vi "InclinometerLogic.vi"   [LabVIEW 2016]
uses:
  InclinometerData.ctl
  InclinometerStates.ctl
  <vilib>/Platform/TimedLoop/XDataNode/timing_clust.ctl
  <vilib>/Platform/TimedLoop/XDataNode/nitl_modes.ctl
  <vilib>/Platform/TimedLoop/XDataNode/wakeup.ctl
  Telemetry/TelemetryFields.ctl
  Telemetry/TelemetryDataTypes.ctl
  Telemetry/TelemetryUpdateModes.ctl
  InclinometerErrorCodes.ctl
  <vilib>/rvi/Emulation/niFpgaSctlEmulationGetInTimedLoop.vi
  <vilib>/rvi/Emulation/niFpgaEmulationReportErrorSimple.vi
  <vilib>/rvi/Emulation/niFpgaGetClockAttributes.vi
  <vilib>/rvi/Emulation/niFpgaCriticalErrorInLSC.vi
  <vilib>/rvi/Emulation/niFpgaEmulationIsFPGAContextNoSignature.vi
  <vilib>/rvi/DataTransferAndStorage/Container/Common/niFpgaContainerGetUniqueNameForEmu.vi
  <vilib>/rvi/Memory/Memory_Emulation/niFpgaMemoryEmulationCacheClearOnFirstRun.vi
  <vilib>/rvi/Memory/Memory_Emulation/nirvimemoryEmulationManagerCache_MakeExclusive.vi
  <vilib>/rvi/Memory/Memory_Emulation/niFpgaMemoryEmulationValidateCache.vi
  <vilib>/rvi/Memory/Memory_Emulation/nirvimemoryEmulationManagerCache_InsertValue.vi
  <vilib>/Utility/error.llb/Clear Errors.vi
  <vilib>/rvi/Memory/Memory_Emulation/nirvimemoryEmulationManagerCache_ReleaseExclusive.vi
  <vilib>/rvi/Memory/Memory_Emulation/nirvimemoryEmulationManagerCache_GetValue.vi
  <vilib>/rvi/Memory/Memory_Emulation/nirvimemoryEmulationManagerCache_SetValue.vi
  <vilib>/rvi/Emulation/niFpgaProcessEmulError.vi
  <vilib>/rvi/errors/niFpgaSetErrorForExecOnDevCompSimple.vi
  <vilib>/rvi/eio/common/nirviEmuReportErrorAndStop.vi
  <vilib>/rvi/FIFO/Fifo_Resource/nirvififoEmulationSetSize.vi
  <vilib>/rvi/FIFO/Fifo_Resource/nirviFifoEmulationQueueMgr.vi
  <instcachedir>/0/nirviFifoEmulationQueueMgr_E5CAEC123FF24DC58D834DCA3CDAA9B5.lvgen/nirviFifoEmulationQueueMgr_E5CAEC123FF24DC58D834DCA3CDAA9B5_004.vi
  <vilib>/rvi/FIFO/Fifo_Resource/nirvififoEmulationDetermineInputValidOut.vi
  <vilib>/rvi/FIFO/Fifo_Resource/nirvififoEmulationCreateLock.vi
  <vilib>/rvi/FIFO/Fifo_Resource/nirvififoEmulationObtainLock.vi
  <vilib>/rvi/FIFO/Fifo_Resource/nirvififoEmulationReleaseLock.vi
  <vilib>/rvi/occurrence/nirviWaitOnOccurrenceBase.vi
  <vilib>/rvi/errors/nirviReportUnexpectedCaseInternalError.vi
  <vilib>/rvi/errors/nirviReportUnexpectedCaseInternalError (U32).vi
  <instcachedir>/0/nirviFifoEmulationQueueMgr_E5CAEC123FF24DC58D834DCA3CDAA9B5.lvgen/nirviFifoEmulationQueueMgr_E5CAEC123FF24DC58D834DCA3CDAA9B5_009.vi
  <instcachedir>/0/nirviFifoEmulationQueueMgr_E5CAEC123FF24DC58D834DCA3CDAA9B5.lvgen/nirviFifoEmulationQueueMgr_E5CAEC123FF24DC58D834DCA3CDAA9B5_002.vi
  <instcachedir>/0/nirviFifoEmulationQueueMgr_E5CAEC123FF24DC58D834DCA3CDAA9B5.lvgen/nirviFifoEmulationQueueMgr_E5CAEC123FF24DC58D834DCA3CDAA9B5_024.vi
  <vilib>/rvi/eio/common/nirviEmuTemplateMethod_errors.vi
  <vilib>/Platform/TimedLoop/XDataNode/XDataNode.xnode
  <vilib>/rvi/DataTransferAndStorage/Container/XNode/niFpgaContainer.xnode
  <vilib>/rvi/DataTransferAndStorage/Register/Emulation/niFpgaRegisterEmulation.vi
  <vilib>/rvi/FIFO/Fifo_Resource/nirvififoEmulationWrite.vi
  <vilib>/rvi/FIFO/Fifo_Resource/nirvififoEmulationRead.vi
  <vilib>/eio/EIONode/EIONode.xnode
  <vilib>/Platform/TimedLoop/XDataNode/XDNodeRunTimeDep.lvlib
types:
  T1 = typedef "InclinometerData.ctl" = cluster{"InclinometerState":T2, "Timestamp":u64, "Timeout":i32, "Angle":u32, "CRC":u16, "Exception":u8}
  T2 = typedef "InclinometerStates.ctl" = enum16{"WaitForTrigger", "ClearRxFIFO", "WaitForClearComplete", "WriteAddress", "WriteFunction", "WriteStartAddress1", "WriteStartAddress0", "WriteAddressCount1", "WriteAddressCount0", "WriteCRC1", "WriteCRC0", "ReadAddress", "ReadFunction", "ReadByteCount", "ReadDataByte1", "ReadDataByte0", "ReadDataByte3", "ReadDataByte2", "ReadCRCByte0", "ReadCRCByte1", "CalculateCRC", "ValidateCRC", "MoveTimestamp", "MoveData", "ClearErrorCode", "ReadExceptionCode", "ReadExceptionCRCByte0", "ReadExceptionCRCByte1", "CalculateExceptionCRC", "ValidateExceptionCRC", "ParseExceptionCode", "ResponseAddressError", "ResponseFunctionCodeError", "ResponseByteCountError", "ResponseCRCError", "ResponseUnknownError", "ResponseTimeoutError", "SensorReportsIllegalFunction", "SensorReportsIllegalDataAddress"}
  T3 = typedef "XDNodeRunTimeDep.lvlib/timing_clust.ctl" = cluster{"Expected End [f-1]":u64, "Actual End [f-1]":u64, "Finished Late? [f-1]":bool, "Expected End [i-1]":u64, "Actual End [i-1]":u64, "Finished Late? [i-1]":bool, "Expected Start [i]":u64, "Actual Start [i]":u64, "Expected Start [f]":u64, "Actual Start [f]":u64, "Source Name":string, "Structure Name":string, "Period":i64, "Deadline":i64, "Offset":i64, "Start":i64, "Priority":i32, "Timeout":i32, "Mode":T4, "Wakeup Reason":T5, "Error":errorcluster, "Source Type":string, "Secondary Source Type":string, "Global End Time":u64, "Global Start Time":u64, "Frame Duration":u64, "Iteration Duration":u64, "Assigned CPU":i32, "I/O Scan Engine Mode":u32}
  T4 = typedef "XDNodeRunTimeDep.lvlib/nitl_modes.ctl" = enum32{"No Change", "Process missed periods, maintain original phase", "Discard missed periods, maintain original phase", "Process missed periods, ignore original phase", "Discard missed periods, ignore original phase"}
  T5 = typedef "XDNodeRunTimeDep.lvlib/wakeup.ctl" = enum32{"Normal", "Aborted", "Asynchronous wakeup", "Timing source error", "Timed loop error", "Timeout"}
  T6 = typedef "TelemetryUpdateModes.ctl" = enum8{"=", "+", "-", "|"}
  T7 = typedef "TelemetryDataTypes.ctl" = enum8{"U8", "U16", "U32", "U64", "I8", "I16", "I32", "I64", "SGL"}
  T8 = typedef "TelemetryFields.ctl" = enum16{"InclinometerErrorCode", "InclinometerTxBytes", "InclinometerRxBytes", "InclinometerTxFrames", "InclinometerRxFrames", "InclinometerTimestamp", "InclinometerAngle", "DisplacementErrorCode", "DisplacementTxBytes", "DisplacementRxBytes", "DisplacementTxFrames", "DisplacementRxFrames", "DisplacementTimestamp", "Displacement1", "Displacement2", "Displacement3", "Displacement4", "Displacement5", "Displacement6", "Displacement7", "Displacement8", "AccelerometerSampleCount", "AccelerometerTimestamp", "AccelerometerRaw1", "AccelerometerRaw2", "AccelerometerRaw3", "AccelerometerRaw4", "AccelerometerRaw5", "AccelerometerRaw6", "AccelerometerRaw7", "AccelerometerRaw8", "AccelerometerEng1", "AccelerometerEng2", "AccelerometerEng3", "AccelerometerEng4", "AccelerometerEng5", "AccelerometerEng6", "AccelerometerEng7", "AccelerometerEng8", "AngularAccelerationX", "AngularAccelerationY", "AngularAccelerationZ"}
  T9 = typedef "InclinometerErrorCodes.ctl" = enum8{"None", "ResponseAddressError", "ResponseFunctionCodeError", "ResponseByteCountError", "ResponseCRCError", "ResponseUnknownError", "ResponseTimeoutError", "SensorReportsIllegalFunction", "SensorReportsIllegalDataAddress"}
  T10 = typedef "TelemetryUpdateData.ctl" = cluster{"DataType":T7, "Mode":T6, "Field":T8, "Data":u64}
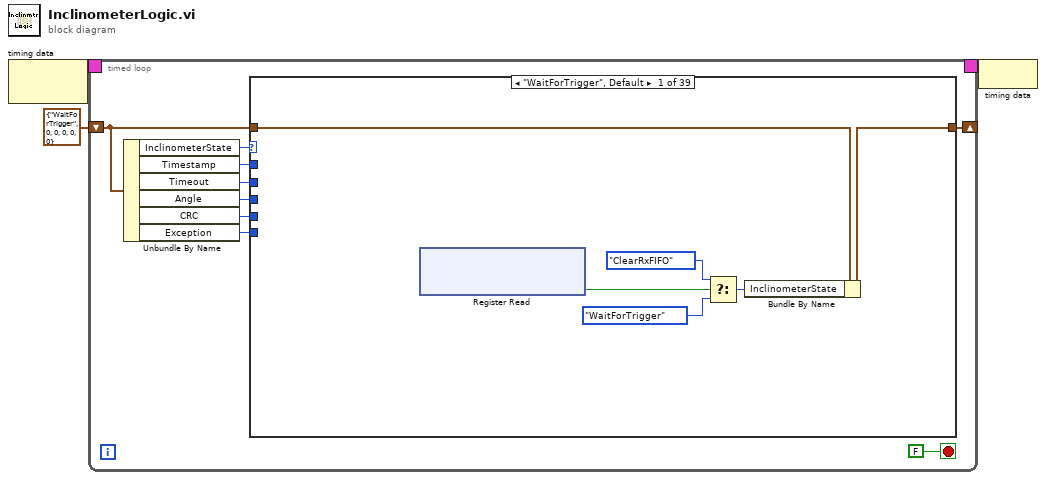
[diagram p0: block diagram]
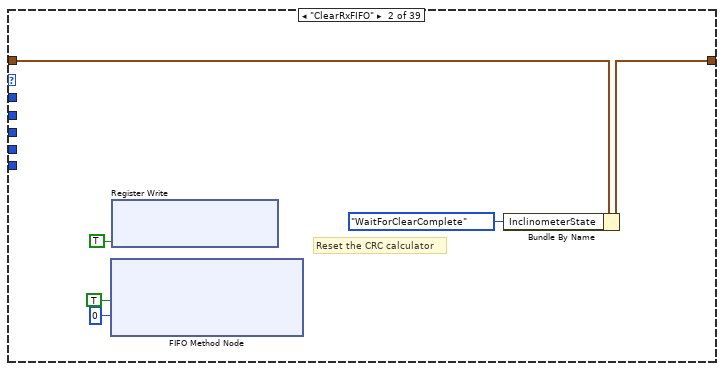
[diagram p2: hidden frame]
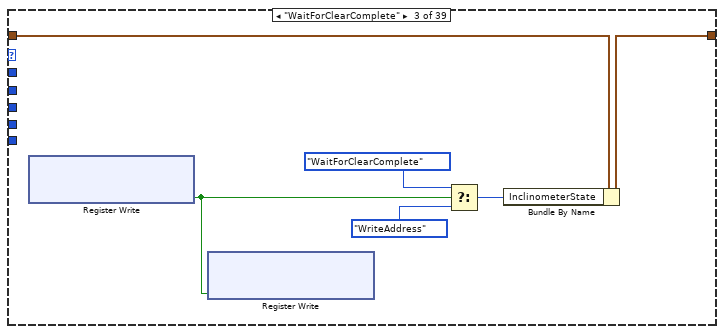
[diagram p3: hidden frame]
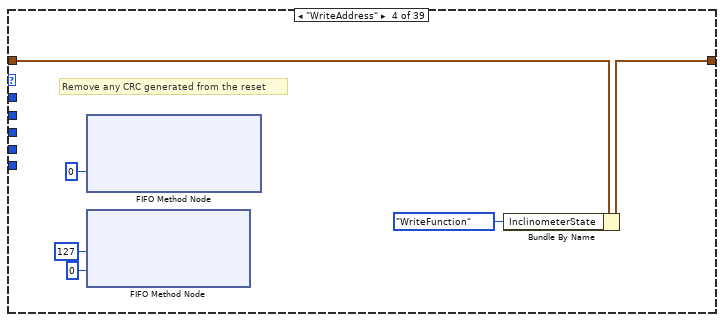
[diagram p4: hidden frame]
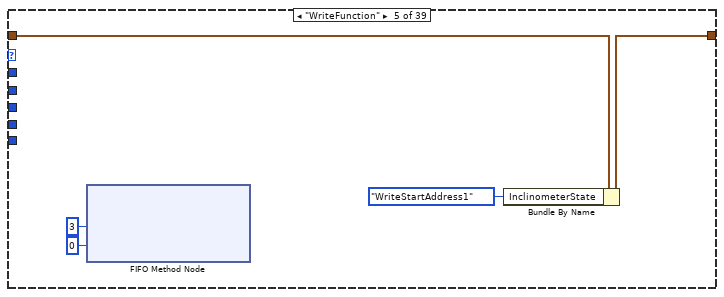
[diagram p5: hidden frame]
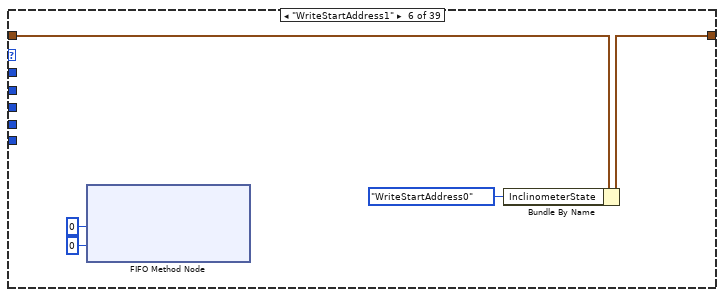
[diagram p6: hidden frame]
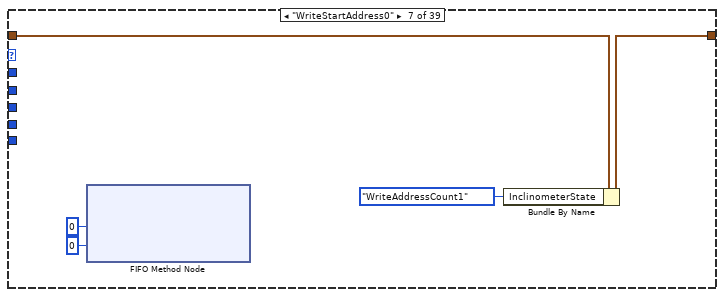
[diagram p7: hidden frame]
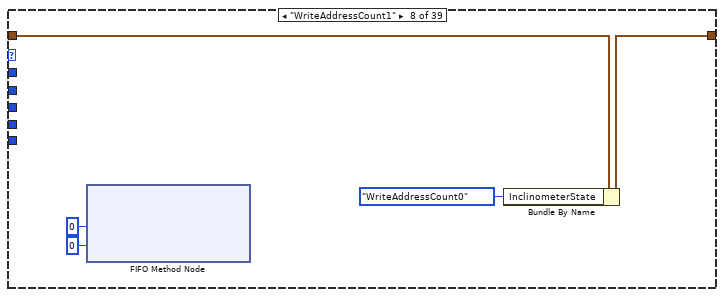
[diagram p8: hidden frame]
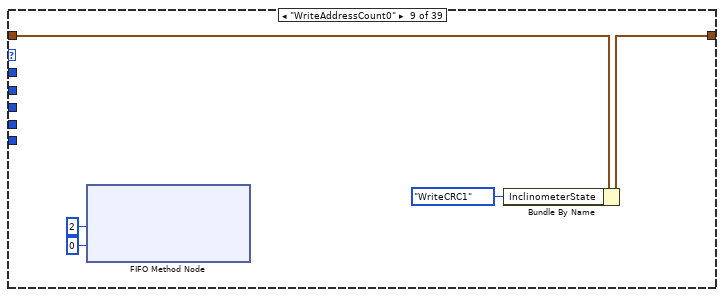
[diagram p9: hidden frame]
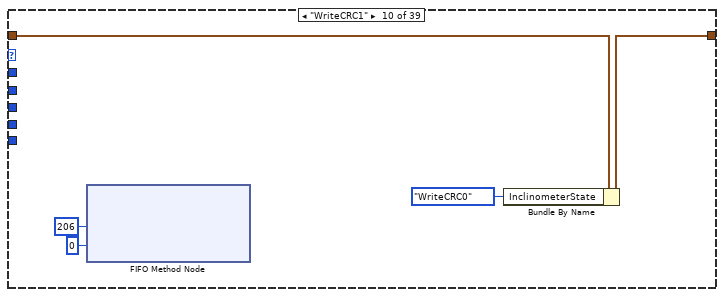
[diagram p10: hidden frame]
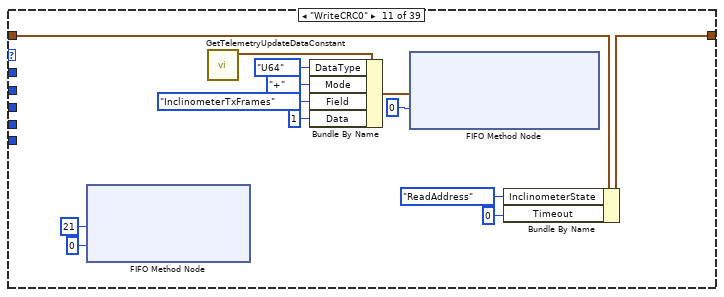
[diagram p11: hidden frame]
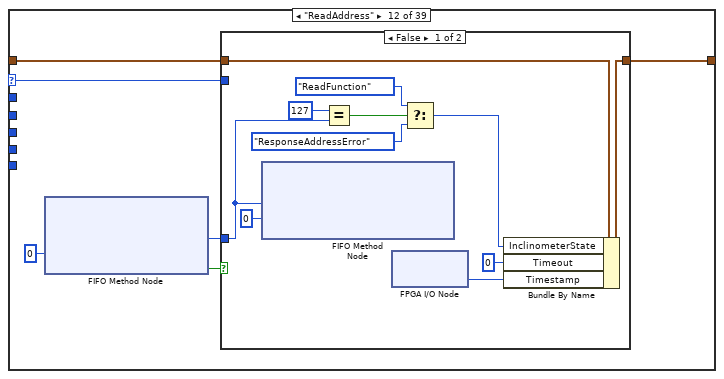
[diagram p12: hidden frame]
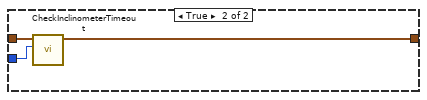
[diagram p13: hidden frame]
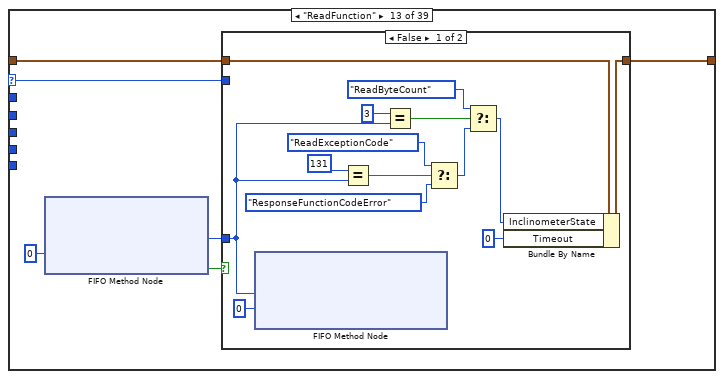
[diagram p14: hidden frame]
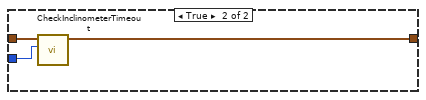
[diagram p15: hidden frame]
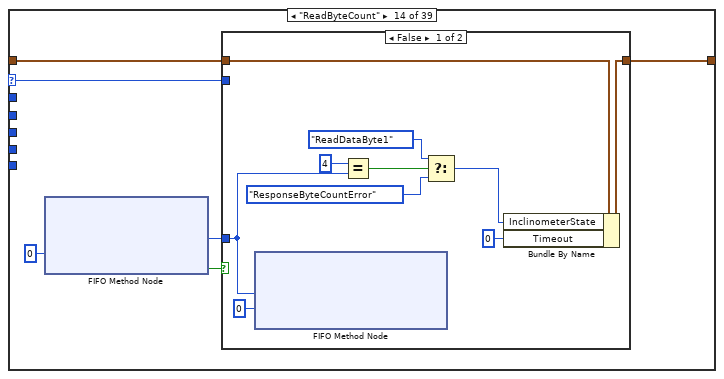
[diagram p16: hidden frame]
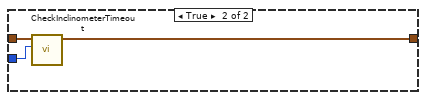
[diagram p17: hidden frame]
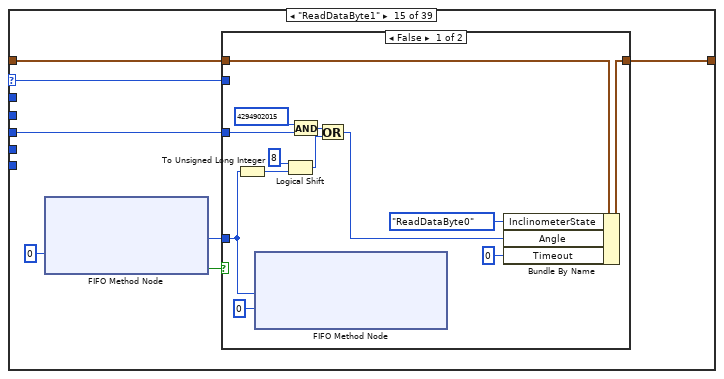
[diagram p18: hidden frame]
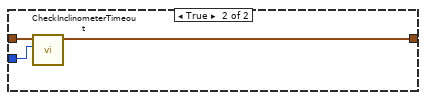
[diagram p19: hidden frame]
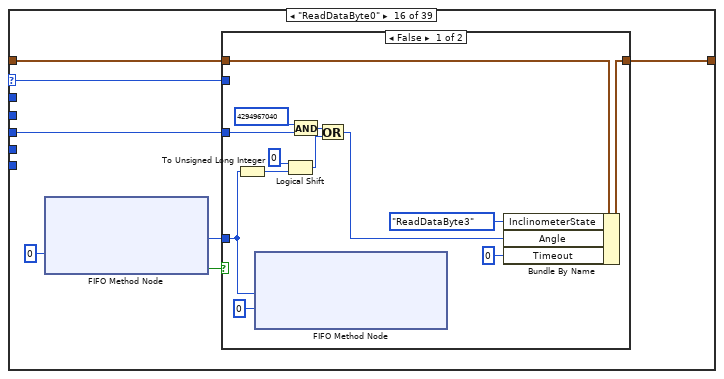
[diagram p20: hidden frame]
diagram:
  n1 = node-c288() -> (w3:T3)  [unwired: 1 in]
  n2 = timed-loop {
    timing: w3 -> [_]
    timing-out: [_] -> w2
    shift-right: [w11] -> _
    shift-left: T1 {"InclinometerState"=enum."WaitForTrigger", "Timestamp"=0, "Timeout"=0, "Angle"=0, "CRC"=0, "Exception"=0} ("InclinometerData") -> [w12]
    stop <- FALSE stop-if-true
    n3 = Unbundle By Name(w12) -> ("InclinometerState"=w10:T2, "Timestamp"=w5:u64, "Timeout"=w9:i32, "Angle"=w8:u32, "CRC"=w7:u16, "Exception"=w4:u8)
    n4 = case shown="\"WaitForTrigger\", Default" w10 {
      selector: w10 -> [_ _ _ _ _ _ _ _ _ _ _ w80 w100 w123 w142 w165 w188 w211 w234 w256 _ _ _ _ _ w335 w357 w379 _ _ _ _ _ _ _ _ _ _ _]
      tunnel: w12 -> [w17 w23 w29 w35 w40 w45 w50 w55 w60 w65 w78 w81 w101 w124 w144 w167 w190 w213 w236 w258 w281 w284 w313 w323 w333 w336 w359 w381 w404 w407 w434 w444 w454 w464 w474 w484 w494 w504 w514]
      tunnel: [w18 w24 w30 w36 w41 w46 w51 w56 w61 w66 w79 w82 w102 w125 w145 w168 w191 w214 w237 w259 w282 w285 w314 w324 w334 w337 w360 w382 w405 w408 w435 w445 w455 w465 w475 w485 w495 w505 w515] -> w11
      tunnel: w9 -> [_ _ _ _ _ _ _ _ _ _ _ _ _ _ _ _ _ _ _ _ _ _ _ _ _ _ _ _ _ _ _ _ _ _ _ _ _ _ _]
      tunnel: w8 -> [_ _ _ _ _ _ _ _ _ _ _ _ _ _ w143 w166 w189 w212 _ _ _ _ _ w315 _ _ _ _ _ _ _ _ _ _ _ _ _ _ _]
      tunnel: w7 -> [_ _ _ _ _ _ _ _ _ _ _ _ _ _ _ _ _ _ w235 w257 _ w283 _ _ _ _ w358 w380 _ w406 _ _ _ _ _ _ _ _ _]
      tunnel: w5 -> [_ _ _ _ _ _ _ _ _ _ _ _ _ _ _ _ _ _ _ _ _ _ w305 _ _ _ _ _ _ _ _ _ _ _ _ _ _ _ _]
      tunnel: w4 -> [_ _ _ _ _ _ _ _ _ _ _ _ _ _ _ _ _ _ _ _ _ _ _ _ _ _ _ _ _ _ w429 _ _ _ _ _ _ _ _]
      frame "WaitForTrigger", Default {
        n5 = xnode ("Register Read")() -> ("Data"=w13:bool)  [unwired: 1 in, 1 out]
        n6 = Select(t=InclinometerStates."ClearRxFIFO" ("InclinometerState"), s=w13, f=InclinometerStates."WaitForTrigger" ("InclinometerState")) -> (s? t:f=w14:T2)
        n7 = Bundle By Name(cluster=w17, "InclinometerState"=w14) -> (w18:T1)
      }
      frame "ClearRxFIFO" {
        # "Reset the CRC calculator"
        n8 = xnode ("FIFO Method Node")("Element"=TRUE, "Timeout"=0) -> ()  [unwired: 1 in, 2 out]
        n9 = xnode ("Register Write")("Data"=TRUE) -> ()  [unwired: 1 in, 1 out]
        n10 = Bundle By Name(cluster=w23, "InclinometerState"=InclinometerStates."WaitForClearComplete") -> (w24:T1)
      }
      frame "WaitForClearComplete" {
        n11 = xnode ("Register Write")() -> ("Data"=w25:bool)  [unwired: 1 in, 1 out]
        n12 = xnode ("Register Write")("Data"=w25) -> ()  [unwired: 1 in, 1 out]
        n13 = Select(t=InclinometerStates."WaitForClearComplete", s=w25, f=InclinometerStates."WriteAddress" ("InclinometerState")) -> (s? t:f=w26:T2)
        n14 = Bundle By Name(cluster=w29, "InclinometerState"=w26) -> (w30:T1)
      }
      frame "WriteAddress" {
        # "Remove any CRC generated from the reset"
        n15 = xnode ("FIFO Method Node")("Timeout"=0) -> ()  [unwired: 1 in, 3 out]
        n16 = xnode ("FIFO Method Node")("Element"=u8 127, "Timeout"=0) -> ()  [unwired: 1 in, 2 out]
        n17 = Bundle By Name(cluster=w35, "InclinometerState"=InclinometerStates."WriteFunction") -> (w36:T1)
      }
      frame "WriteFunction" {
        n18 = xnode ("FIFO Method Node")("Element"=u8 3, "Timeout"=0) -> ()  [unwired: 1 in, 2 out]
        n19 = Bundle By Name(cluster=w40, "InclinometerState"=InclinometerStates."WriteStartAddress1") -> (w41:T1)
      }
      frame "WriteStartAddress1" {
        n20 = xnode ("FIFO Method Node")("Element"=u8 0, "Timeout"=0) -> ()  [unwired: 1 in, 2 out]
        n21 = Bundle By Name(cluster=w45, "InclinometerState"=InclinometerStates."WriteStartAddress0") -> (w46:T1)
      }
      frame "WriteStartAddress0" {
        n22 = xnode ("FIFO Method Node")("Element"=u8 0, "Timeout"=0) -> ()  [unwired: 1 in, 2 out]
        n23 = Bundle By Name(cluster=w50, "InclinometerState"=InclinometerStates."WriteAddressCount1") -> (w51:T1)
      }
      frame "WriteAddressCount1" {
        n24 = xnode ("FIFO Method Node")("Element"=u8 0, "Timeout"=0) -> ()  [unwired: 1 in, 2 out]
        n25 = Bundle By Name(cluster=w55, "InclinometerState"=InclinometerStates."WriteAddressCount0") -> (w56:T1)
      }
      frame "WriteAddressCount0" {
        n26 = xnode ("FIFO Method Node")("Element"=u8 2, "Timeout"=0) -> ()  [unwired: 1 in, 2 out]
        n27 = Bundle By Name(cluster=w60, "InclinometerState"=InclinometerStates."WriteCRC1") -> (w61:T1)
      }
      frame "WriteCRC1" {
        n28 = xnode ("FIFO Method Node")("Element"=u8 206, "Timeout"=0) -> ()  [unwired: 1 in, 2 out]
        n29 = Bundle By Name(cluster=w65, "InclinometerState"=InclinometerStates."WriteCRC0") -> (w66:T1)
      }
      frame "WriteCRC0" {
        n30 = xnode ("FIFO Method Node")("Element"=u8 21, "Timeout"=0) -> ()  [unwired: 1 in, 2 out]
        n31 = call "GetTelemetryUpdateDataConstant.vi"() -> ("TelemetryUpdateData"=w71:T10)  [unwired: 11 in]
        n32 = Bundle By Name(cluster=w71, "DataType"=TelemetryDataTypes."U64" ("TelemetryDataTypes"), "Mode"=TelemetryUpdateModes."+" ("TelemetryUpdateModes"), "Field"=TelemetryFields."InclinometerTxFrames", "Data"=u64 1) -> (w67:T10)
        n33 = xnode ("FIFO Method Node")("Element"=w67, "Timeout"=0) -> ()  [unwired: 1 in, 2 out]
        n34 = Bundle By Name(cluster=w78, "InclinometerState"=InclinometerStates."ReadAddress", "Timeout"=0) -> (w79:T1)
      }
      frame "ReadAddress" {
        n35 = xnode ("FIFO Method Node")("Timeout"=0) -> ("Element"=w83:u8, "Timed Out?"=w84:bool)  [unwired: 1 in, 1 out]
        n36 = case shown="False" w84 {
          tunnel: w83 -> [w93 _]
          tunnel: [w95 w98] -> w82
          tunnel: w81 -> [w96 w99]
          tunnel: w80 -> [_ w97]
          frame False {
            n37 = xnode ("FIFO Method Node")("Element"=w93, "Timeout"=0) -> ()  [unwired: 1 in, 2 out]
            n38 = Equal?(x=u8 127, y=w93) -> (x = y?=w91:bool)
            n39 = xnode "FPGA I/O Node"() -> ("Time"=w86:u64)  [unwired: 1 in, 1 out]
            n40 = Select(t=InclinometerStates."ReadFunction" ("InclinometerState"), s=w91, f=InclinometerStates."ResponseAddressError" ("InclinometerState")) -> (s? t:f=w88:T2)
            n41 = Bundle By Name(cluster=w96, "InclinometerState"=w88, "Timeout"=0, "Timestamp"=w86) -> (w95:T1)
          }
          frame True {
            n42 = call "CheckInclinometerTimeout.vi"("StateIfNoTimeout"=w97, "InclinometerData in"=w99) -> ("InclinometerData out"=w98:T1)  [unwired: 9 in]
          }
        }
      }
      frame "ReadFunction" {
        n43 = xnode ("FIFO Method Node")("Timeout"=0) -> ("Element"=w103:u8, "Timed Out?"=w104:bool)  [unwired: 1 in, 1 out]
        n44 = case shown="False" w104 {
          tunnel: w103 -> [w111 _]
          tunnel: [w118 w121] -> w102
          tunnel: w101 -> [w119 w122]
          tunnel: w100 -> [_ w120]
          frame False {
            n45 = xnode ("FIFO Method Node")("Element"=w111, "Timeout"=0) -> ()  [unwired: 1 in, 2 out]
            n46 = Equal?(x=u8 131, y=w111) -> (x = y?=w110:bool)
            n47 = Equal?(x=u8 3, y=w111) -> (x = y?=w115:bool)
            n48 = Select(t=InclinometerStates."ReadExceptionCode" ("InclinometerState"), s=w110, f=InclinometerStates."ResponseFunctionCodeError" ("InclinometerState")) -> (s? t:f=w113:T2)
            n49 = Select(t=InclinometerStates."ReadByteCount" ("InclinometerState"), s=w115, f=w113) -> (s? t:f=w107:T2)
            n50 = Bundle By Name(cluster=w119, "InclinometerState"=w107, "Timeout"=0) -> (w118:T1)
          }
          frame True {
            n51 = call "CheckInclinometerTimeout.vi"("StateIfNoTimeout"=w120, "InclinometerData in"=w122) -> ("InclinometerData out"=w121:T1)  [unwired: 9 in]
          }
        }
      }
      frame "ReadByteCount" {
        n52 = xnode ("FIFO Method Node")("Timeout"=0) -> ("Element"=w126:u8, "Timed Out?"=w127:bool)  [unwired: 1 in, 1 out]
        n53 = case shown="False" w127 {
          tunnel: w126 -> [w135 _]
          tunnel: [w137 w140] -> w125
          tunnel: w124 -> [w138 w141]
          tunnel: w123 -> [_ w139]
          frame False {
            n54 = xnode ("FIFO Method Node")("Element"=w135, "Timeout"=0) -> ()  [unwired: 1 in, 2 out]
            n55 = Equal?(x=u8 4, y=w135) -> (x = y?=w133:bool)
            n56 = Select(t=InclinometerStates."ReadDataByte1" ("InclinometerState"), s=w133, f=InclinometerStates."ResponseByteCountError" ("InclinometerState")) -> (s? t:f=w130:T2)
            n57 = Bundle By Name(cluster=w138, "InclinometerState"=w130, "Timeout"=0) -> (w137:T1)
          }
          frame True {
            n58 = call "CheckInclinometerTimeout.vi"("StateIfNoTimeout"=w139, "InclinometerData in"=w141) -> ("InclinometerData out"=w140:T1)  [unwired: 9 in]
          }
        }
      }
      frame "ReadDataByte1" {
        n59 = xnode ("FIFO Method Node")("Timeout"=0) -> ("Element"=w146:u8, "Timed Out?"=w147:bool)  [unwired: 1 in, 1 out]
        n60 = case shown="False" w147 {
          tunnel: w146 -> [w152 _]
          tunnel: [w160 w163] -> w145
          tunnel: w144 -> [w161 w164]
          tunnel: w143 -> [w156 _]
          tunnel: w142 -> [_ w162]
          frame False {
            n61 = To Unsigned Long Integer(number=w152) -> (unsigned 32bit integer=w151:u32)
            n62 = xnode ("FIFO Method Node")("Element"=w152, "Timeout"=0) -> ()  [unwired: 1 in, 2 out]
            n63 = Logical Shift(y=i16 8, x=w151) -> (x << y=w154:u32)
            n64 = And(x=u32 4294902015, y=w156) -> (x .and. y?=w153:u32)
            n65 = Or(x=w153, y=w154) -> (x .or. y?=w150:u32)
            n66 = Bundle By Name(cluster=w161, "InclinometerState"=InclinometerStates."ReadDataByte0", "Angle"=w150, "Timeout"=0) -> (w160:T1)
          }
          frame True {
            n67 = call "CheckInclinometerTimeout.vi"("StateIfNoTimeout"=w162, "InclinometerData in"=w164) -> ("InclinometerData out"=w163:T1)  [unwired: 9 in]
          }
        }
      }
      frame "ReadDataByte0" {
        n68 = xnode ("FIFO Method Node")("Timeout"=0) -> ("Element"=w169:u8, "Timed Out?"=w170:bool)  [unwired: 1 in, 1 out]
        n69 = case shown="False" w170 {
          tunnel: w169 -> [w175 _]
          tunnel: [w183 w186] -> w168
          tunnel: w167 -> [w184 w187]
          tunnel: w166 -> [w179 _]
          tunnel: w165 -> [_ w185]
          frame False {
            n70 = To Unsigned Long Integer(number=w175) -> (unsigned 32bit integer=w174:u32)
            n71 = xnode ("FIFO Method Node")("Element"=w175, "Timeout"=0) -> ()  [unwired: 1 in, 2 out]
            n72 = Logical Shift(y=i16 0, x=w174) -> (x << y=w177:u32)
            n73 = And(x=u32 4294967040, y=w179) -> (x .and. y?=w176:u32)
            n74 = Or(x=w176, y=w177) -> (x .or. y?=w173:u32)
            n75 = Bundle By Name(cluster=w184, "InclinometerState"=InclinometerStates."ReadDataByte3", "Angle"=w173, "Timeout"=0) -> (w183:T1)
          }
          frame True {
            n76 = call "CheckInclinometerTimeout.vi"("StateIfNoTimeout"=w185, "InclinometerData in"=w187) -> ("InclinometerData out"=w186:T1)  [unwired: 9 in]
          }
        }
      }
      frame "ReadDataByte3" {
        n77 = xnode ("FIFO Method Node")("Timeout"=0) -> ("Element"=w192:u8, "Timed Out?"=w193:bool)  [unwired: 1 in, 1 out]
        n78 = case shown="False" w193 {
          tunnel: w192 -> [w198 _]
          tunnel: [w206 w209] -> w191
          tunnel: w190 -> [w207 w210]
          tunnel: w189 -> [w202 _]
          tunnel: w188 -> [_ w208]
          frame False {
            n79 = To Unsigned Long Integer(number=w198) -> (unsigned 32bit integer=w197:u32)
            n80 = xnode ("FIFO Method Node")("Element"=w198, "Timeout"=0) -> ()  [unwired: 1 in, 2 out]
            n81 = Logical Shift(y=i16 24, x=w197) -> (x << y=w200:u32)
            n82 = And(x=u32 16777215, y=w202) -> (x .and. y?=w199:u32)
            n83 = Or(x=w199, y=w200) -> (x .or. y?=w196:u32)
            n84 = Bundle By Name(cluster=w207, "InclinometerState"=InclinometerStates."ReadDataByte2", "Angle"=w196, "Timeout"=0) -> (w206:T1)
          }
          frame True {
            n85 = call "CheckInclinometerTimeout.vi"("StateIfNoTimeout"=w208, "InclinometerData in"=w210) -> ("InclinometerData out"=w209:T1)  [unwired: 9 in]
          }
        }
      }
      frame "ReadDataByte2" {
        n86 = xnode ("FIFO Method Node")("Timeout"=0) -> ("Element"=w215:u8, "Timed Out?"=w216:bool)  [unwired: 1 in, 1 out]
        n87 = case shown="False" w216 {
          tunnel: w215 -> [w221 _]
          tunnel: [w229 w232] -> w214
          tunnel: w213 -> [w230 w233]
          tunnel: w212 -> [w225 _]
          tunnel: w211 -> [_ w231]
          frame False {
            n88 = To Unsigned Long Integer(number=w221) -> (unsigned 32bit integer=w220:u32)
            n89 = xnode ("FIFO Method Node")("Element"=w221, "Timeout"=0) -> ()  [unwired: 1 in, 2 out]
            n90 = Logical Shift(y=i16 16, x=w220) -> (x << y=w223:u32)
            n91 = And(x=u32 4278255615, y=w225) -> (x .and. y?=w222:u32)
            n92 = Or(x=w222, y=w223) -> (x .or. y?=w219:u32)
            n93 = Bundle By Name(cluster=w230, "InclinometerState"=InclinometerStates."ReadCRCByte0", "Angle"=w219, "Timeout"=0) -> (w229:T1)
          }
          frame True {
            n94 = call "CheckInclinometerTimeout.vi"("StateIfNoTimeout"=w231, "InclinometerData in"=w233) -> ("InclinometerData out"=w232:T1)  [unwired: 9 in]
          }
        }
      }
      frame "ReadCRCByte0" {
        n95 = xnode ("FIFO Method Node")("Timeout"=0) -> ("Element"=w238:u8, "Timed Out?"=w239:bool)  [unwired: 1 in, 1 out]
        n96 = case shown="False" w239 {
          tunnel: w238 -> [w245 _]
          tunnel: [w251 w254] -> w237
          tunnel: w236 -> [w252 w255]
          tunnel: w235 -> [w242 _]
          tunnel: w234 -> [_ w253]
          frame False {
            n97 = To Unsigned Word Integer(number=w245) -> (unsigned 16bit integer=w244:u16)
            n98 = Logical Shift(y=i16 0, x=w244) -> (x << y=w247:u16)
            n99 = And(x=u16 65280, y=w242) -> (x .and. y?=w246:u16)
            n100 = Or(x=w246, y=w247) -> (x .or. y?=w243:u16)
            n101 = Bundle By Name(cluster=w252, "InclinometerState"=InclinometerStates."ReadCRCByte1", "CRC"=w243, "Timeout"=0) -> (w251:T1)
          }
          frame True {
            n102 = call "CheckInclinometerTimeout.vi"("StateIfNoTimeout"=w253, "InclinometerData in"=w255) -> ("InclinometerData out"=w254:T1)  [unwired: 9 in]
          }
        }
      }
      frame "ReadCRCByte1" {
        n103 = xnode ("FIFO Method Node")("Timeout"=0) -> ("Element"=w260:u8, "Timed Out?"=w261:bool)  [unwired: 1 in, 1 out]
        n104 = case shown="False" w261 {
          tunnel: w260 -> [w267 _]
          tunnel: [w273 w276] -> w259
          tunnel: w258 -> [w274 w277]
          tunnel: w257 -> [w264 _]
          tunnel: w256 -> [_ w275]
          frame False {
            n105 = To Unsigned Word Integer(number=w267) -> (unsigned 16bit integer=w266:u16)
            n106 = Logical Shift(y=i16 8, x=w266) -> (x << y=w269:u16)
            n107 = And(x=u16 255, y=w264) -> (x .and. y?=w268:u16)
            n108 = Or(x=w268, y=w269) -> (x .or. y?=w265:u16)
            n109 = Bundle By Name(cluster=w274, "InclinometerState"=InclinometerStates."CalculateCRC", "CRC"=w265, "Timeout"=0) -> (w273:T1)
          }
          frame True {
            n110 = call "CheckInclinometerTimeout.vi"("StateIfNoTimeout"=w275, "InclinometerData in"=w277) -> ("InclinometerData out"=w276:T1)  [unwired: 9 in]
          }
        }
      }
      frame "CalculateCRC" {
        n111 = xnode ("FIFO Method Node")("Element"=TRUE, "Timeout"=0) -> ()  [unwired: 1 in, 2 out]
        n112 = Bundle By Name(cluster=w281, "InclinometerState"=InclinometerStates."ValidateCRC") -> (w282:T1)
      }
      frame "ValidateCRC" {
        n113 = xnode ("FIFO Method Node")("Timeout"=0) -> ("Element"=w286:u16, "Timed Out?"=w287:bool)  [unwired: 1 in, 1 out]
        n114 = case shown="False" w287 {
          tunnel: w286 -> [w296 _]
          tunnel: [w302 w304] -> w285
          tunnel: w284 -> [w303 w304]
          tunnel: w283 -> [w297 _]
          frame False {
            n115 = call "GetTelemetryUpdateDataConstant.vi"() -> ("TelemetryUpdateData"=w293:T10)  [unwired: 11 in]
            n116 = Equal?(x=w297, y=w296) -> (x = y?=w301:bool)
            n117 = Bundle By Name(cluster=w293, "DataType"=TelemetryDataTypes."U64" ("TelemetryDataTypes"), "Mode"=TelemetryUpdateModes."+" ("TelemetryUpdateModes"), "Field"=TelemetryFields."InclinometerRxFrames", "Data"=u64 1) -> (w289:T10)
            n118 = Select(t=InclinometerStates."MoveTimestamp" ("InclinometerState"), s=w301, f=InclinometerStates."ResponseCRCError" ("InclinometerState")) -> (s? t:f=w298:T2)
            n119 = xnode ("FIFO Method Node")("Element"=w289, "Timeout"=0) -> ()  [unwired: 1 in, 2 out]
            n120 = Bundle By Name(cluster=w303, "InclinometerState"=w298) -> (w302:T1)
          }
          frame True {
          }
        }
      }
      frame "MoveTimestamp" {
        n121 = call "GetTelemetryUpdateDataConstant.vi"() -> ("TelemetryUpdateData"=w310:T10)  [unwired: 11 in]
        n122 = Bundle By Name(cluster=w310, "DataType"=TelemetryDataTypes."U64" ("TelemetryDataTypes"), "Mode"=TelemetryUpdateModes."=" ("TelemetryUpdateModes"), "Field"=TelemetryFields."InclinometerTimestamp", "Data"=w305) -> (w306:T10)
        n123 = xnode ("FIFO Method Node")("Element"=w306, "Timeout"=0) -> ()  [unwired: 1 in, 2 out]
        n124 = Bundle By Name(cluster=w313, "InclinometerState"=InclinometerStates."MoveData") -> (w314:T1)
      }
      frame "MoveData" {
        n125 = call "GetTelemetryUpdateDataConstant.vi"() -> ("TelemetryUpdateData"=w320:T10)  [unwired: 11 in]
        n126 = Bundle By Name(cluster=w320, "DataType"=TelemetryDataTypes."U32" ("TelemetryDataTypes"), "Mode"=TelemetryUpdateModes."=" ("TelemetryUpdateModes"), "Field"=TelemetryFields."InclinometerAngle", "Data"=w315) -> (w316:T10)
        n127 = xnode ("FIFO Method Node")("Element"=w316, "Timeout"=0) -> ()  [unwired: 1 in, 2 out]
        n128 = Bundle By Name(cluster=w323, "InclinometerState"=InclinometerStates."ClearErrorCode") -> (w324:T1)
      }
      frame "ClearErrorCode" {
        n129 = call "GetTelemetryUpdateDataConstant.vi"() -> ("TelemetryUpdateData"=w330:T10)  [unwired: 11 in]
        n130 = Bundle By Name(cluster=w330, "DataType"=TelemetryDataTypes."U8" ("TelemetryDataTypes"), "Mode"=TelemetryUpdateModes."=" ("TelemetryUpdateModes"), "Field"=TelemetryFields."InclinometerErrorCode", "Data"=InclinometerErrorCodes."None" ("InclinometerErrorCodes")) -> (w326:T10)
        n131 = xnode ("FIFO Method Node")("Element"=w326, "Timeout"=0) -> ()  [unwired: 1 in, 2 out]
        n132 = Bundle By Name(cluster=w333, "InclinometerState"=InclinometerStates."WaitForTrigger") -> (w334:T1)
      }
      frame "ReadExceptionCode" {
        n133 = xnode ("FIFO Method Node")("Timeout"=0) -> ("Element"=w338:u8, "Timed Out?"=w339:bool)  [unwired: 1 in, 1 out]
        n134 = case shown="False" w339 {
          tunnel: w338 -> [w341 _]
          tunnel: [w352 w355] -> w337
          tunnel: w336 -> [w353 w356]
          tunnel: w335 -> [_ w354]
          frame False {
            n135 = xnode ("FIFO Method Node")("Element"=w341, "Timeout"=0) -> ()  [unwired: 1 in, 2 out]
            n136 = Equal?(x=u8 1, y=w341) -> (x = y?=w344:bool)
            n137 = Equal?(x=u8 2, y=w341) -> (x = y?=w343:bool)
            n138 = Or(x=w344, y=w343) -> (x .or. y?=w342:bool)
            n139 = Select(t=InclinometerStates."ReadExceptionCRCByte0" ("InclinometerState"), s=w342, f=InclinometerStates."ResponseUnknownError" ("InclinometerState")) -> (s? t:f=w347:T2)
            n140 = Bundle By Name(cluster=w353, "InclinometerState"=w347, "Timeout"=0, "Exception"=w341) -> (w352:T1)
          }
          frame True {
            n141 = call "CheckInclinometerTimeout.vi"("StateIfNoTimeout"=w354, "InclinometerData in"=w356) -> ("InclinometerData out"=w355:T1)  [unwired: 9 in]
          }
        }
      }
      frame "ReadExceptionCRCByte0" {
        n142 = xnode ("FIFO Method Node")("Timeout"=0) -> ("Element"=w361:u8, "Timed Out?"=w362:bool)  [unwired: 1 in, 1 out]
        n143 = case shown="False" w362 {
          tunnel: w361 -> [w368 _]
          tunnel: [w374 w377] -> w360
          tunnel: w359 -> [w375 w378]
          tunnel: w358 -> [w365 _]
          tunnel: w357 -> [_ w376]
          frame False {
            n144 = To Unsigned Word Integer(number=w368) -> (unsigned 16bit integer=w367:u16)
            n145 = Logical Shift(y=i16 0, x=w367) -> (x << y=w370:u16)
            n146 = And(x=u16 65280, y=w365) -> (x .and. y?=w369:u16)
            n147 = Or(x=w369, y=w370) -> (x .or. y?=w366:u16)
            n148 = Bundle By Name(cluster=w375, "InclinometerState"=InclinometerStates."ReadExceptionCRCByte1", "CRC"=w366, "Timeout"=0) -> (w374:T1)
          }
          frame True {
            n149 = call "CheckInclinometerTimeout.vi"("StateIfNoTimeout"=w376, "InclinometerData in"=w378) -> ("InclinometerData out"=w377:T1)  [unwired: 9 in]
          }
        }
      }
      frame "ReadExceptionCRCByte1" {
        n150 = xnode ("FIFO Method Node")("Timeout"=0) -> ("Element"=w383:u8, "Timed Out?"=w384:bool)  [unwired: 1 in, 1 out]
        n151 = case shown="False" w384 {
          tunnel: w383 -> [w390 _]
          tunnel: [w396 w399] -> w382
          tunnel: w381 -> [w397 w400]
          tunnel: w380 -> [w387 _]
          tunnel: w379 -> [_ w398]
          frame False {
            n152 = To Unsigned Word Integer(number=w390) -> (unsigned 16bit integer=w389:u16)
            n153 = Logical Shift(y=i16 8, x=w389) -> (x << y=w392:u16)
            n154 = And(x=u16 255, y=w387) -> (x .and. y?=w391:u16)
            n155 = Or(x=w391, y=w392) -> (x .or. y?=w388:u16)
            n156 = Bundle By Name(cluster=w397, "InclinometerState"=InclinometerStates."CalculateExceptionCRC", "CRC"=w388, "Timeout"=0) -> (w396:T1)
          }
          frame True {
            n157 = call "CheckInclinometerTimeout.vi"("StateIfNoTimeout"=w398, "InclinometerData in"=w400) -> ("InclinometerData out"=w399:T1)  [unwired: 9 in]
          }
        }
      }
      frame "CalculateExceptionCRC" {
        n158 = xnode ("FIFO Method Node")("Element"=TRUE, "Timeout"=0) -> ()  [unwired: 1 in, 2 out]
        n159 = Bundle By Name(cluster=w404, "InclinometerState"=InclinometerStates."ValidateExceptionCRC") -> (w405:T1)
      }
      frame "ValidateExceptionCRC" {
        n160 = xnode ("FIFO Method Node")("Timeout"=0) -> ("Element"=w409:u16, "Timed Out?"=w410:bool)  [unwired: 1 in, 1 out]
        n161 = case shown="False" w410 {
          tunnel: w409 -> [w419 _]
          tunnel: [w425 w427] -> w408
          tunnel: w407 -> [w426 w427]
          tunnel: w406 -> [w420 _]
          frame False {
            n162 = call "GetTelemetryUpdateDataConstant.vi"() -> ("TelemetryUpdateData"=w417:T10)  [unwired: 11 in]
            n163 = Equal?(x=w420, y=w419) -> (x = y?=w424:bool)
            n164 = Bundle By Name(cluster=w417, "DataType"=TelemetryDataTypes."U64" ("TelemetryDataTypes"), "Mode"=TelemetryUpdateModes."+" ("TelemetryUpdateModes"), "Field"=TelemetryFields."InclinometerRxFrames", "Data"=u64 1) -> (w413:T10)
            n165 = Select(t=InclinometerStates."ParseExceptionCode" ("InclinometerState"), s=w424, f=InclinometerStates."ResponseCRCError" ("InclinometerState")) -> (s? t:f=w421:T2)
            n166 = xnode ("FIFO Method Node")("Element"=w413, "Timeout"=0) -> ()  [unwired: 1 in, 2 out]
            n167 = Bundle By Name(cluster=w426, "InclinometerState"=w421) -> (w425:T1)
          }
          frame True {
          }
        }
      }
      frame "ParseExceptionCode" {
        n168 = Equal?(x=w429, y=u8 1) -> (x = y?=w433:bool)
        n169 = Select(t=InclinometerStates."SensorReportsIllegalFunction" ("InclinometerState"), s=w433, f=InclinometerStates."SensorReportsIllegalDataAddress" ("InclinometerState")) -> (s? t:f=w430:T2)
        n170 = Bundle By Name(cluster=w434, "InclinometerState"=w430) -> (w435:T1)
      }
      frame "ResponseAddressError" {
        n171 = call "GetTelemetryUpdateDataConstant.vi"() -> ("TelemetryUpdateData"=w441:T10)  [unwired: 11 in]
        n172 = Bundle By Name(cluster=w441, "DataType"=TelemetryDataTypes."U8" ("TelemetryDataTypes"), "Mode"=TelemetryUpdateModes."=" ("TelemetryUpdateModes"), "Field"=TelemetryFields."InclinometerErrorCode", "Data"=InclinometerErrorCodes."ResponseAddressError" ("InclinometerErrorCodes")) -> (w436:T10)
        n173 = xnode ("FIFO Method Node")("Element"=w436, "Timeout"=0) -> ()  [unwired: 1 in, 2 out]
        n174 = Bundle By Name(cluster=w444, "InclinometerState"=InclinometerStates."WaitForTrigger") -> (w445:T1)
      }
      frame "ResponseFunctionCodeError" {
        n175 = call "GetTelemetryUpdateDataConstant.vi"() -> ("TelemetryUpdateData"=w451:T10)  [unwired: 11 in]
        n176 = Bundle By Name(cluster=w451, "DataType"=TelemetryDataTypes."U8" ("TelemetryDataTypes"), "Mode"=TelemetryUpdateModes."=" ("TelemetryUpdateModes"), "Field"=TelemetryFields."InclinometerErrorCode", "Data"=InclinometerErrorCodes."ResponseFunctionCodeError" ("InclinometerErrorCodes")) -> (w446:T10)
        n177 = xnode ("FIFO Method Node")("Element"=w446, "Timeout"=0) -> ()  [unwired: 1 in, 2 out]
        n178 = Bundle By Name(cluster=w454, "InclinometerState"=InclinometerStates."WaitForTrigger") -> (w455:T1)
      }
      frame "ResponseByteCountError" {
        n179 = call "GetTelemetryUpdateDataConstant.vi"() -> ("TelemetryUpdateData"=w461:T10)  [unwired: 11 in]
        n180 = Bundle By Name(cluster=w461, "DataType"=TelemetryDataTypes."U8" ("TelemetryDataTypes"), "Mode"=TelemetryUpdateModes."=" ("TelemetryUpdateModes"), "Field"=TelemetryFields."InclinometerErrorCode", "Data"=InclinometerErrorCodes."ResponseByteCountError" ("InclinometerErrorCodes")) -> (w456:T10)
        n181 = xnode ("FIFO Method Node")("Element"=w456, "Timeout"=0) -> ()  [unwired: 1 in, 2 out]
        n182 = Bundle By Name(cluster=w464, "InclinometerState"=InclinometerStates."WaitForTrigger") -> (w465:T1)
      }
      frame "ResponseCRCError" {
        n183 = call "GetTelemetryUpdateDataConstant.vi"() -> ("TelemetryUpdateData"=w471:T10)  [unwired: 11 in]
        n184 = Bundle By Name(cluster=w471, "DataType"=TelemetryDataTypes."U8" ("TelemetryDataTypes"), "Mode"=TelemetryUpdateModes."=" ("TelemetryUpdateModes"), "Field"=TelemetryFields."InclinometerErrorCode", "Data"=InclinometerErrorCodes."ResponseCRCError" ("InclinometerErrorCodes")) -> (w466:T10)
        n185 = xnode ("FIFO Method Node")("Element"=w466, "Timeout"=0) -> ()  [unwired: 1 in, 2 out]
        n186 = Bundle By Name(cluster=w474, "InclinometerState"=InclinometerStates."WaitForTrigger") -> (w475:T1)
      }
      frame "ResponseUnknownError" {
        n187 = call "GetTelemetryUpdateDataConstant.vi"() -> ("TelemetryUpdateData"=w481:T10)  [unwired: 11 in]
        n188 = Bundle By Name(cluster=w481, "DataType"=TelemetryDataTypes."U8" ("TelemetryDataTypes"), "Mode"=TelemetryUpdateModes."=" ("TelemetryUpdateModes"), "Field"=TelemetryFields."InclinometerErrorCode", "Data"=InclinometerErrorCodes."ResponseUnknownError" ("InclinometerErrorCodes")) -> (w476:T10)
        n189 = xnode ("FIFO Method Node")("Element"=w476, "Timeout"=0) -> ()  [unwired: 1 in, 2 out]
        n190 = Bundle By Name(cluster=w484, "InclinometerState"=InclinometerStates."WaitForTrigger") -> (w485:T1)
      }
      frame "ResponseTimeoutError" {
        n191 = call "GetTelemetryUpdateDataConstant.vi"() -> ("TelemetryUpdateData"=w491:T10)  [unwired: 11 in]
        n192 = Bundle By Name(cluster=w491, "DataType"=TelemetryDataTypes."U8" ("TelemetryDataTypes"), "Mode"=TelemetryUpdateModes."=" ("TelemetryUpdateModes"), "Field"=TelemetryFields."InclinometerErrorCode", "Data"=InclinometerErrorCodes."ResponseTimeoutError" ("InclinometerErrorCodes")) -> (w486:T10)
        n193 = xnode ("FIFO Method Node")("Element"=w486, "Timeout"=0) -> ()  [unwired: 1 in, 2 out]
        n194 = Bundle By Name(cluster=w494, "InclinometerState"=InclinometerStates."WaitForTrigger") -> (w495:T1)
      }
      frame "SensorReportsIllegalFunction" {
        n195 = call "GetTelemetryUpdateDataConstant.vi"() -> ("TelemetryUpdateData"=w501:T10)  [unwired: 11 in]
        n196 = Bundle By Name(cluster=w501, "DataType"=TelemetryDataTypes."U8" ("TelemetryDataTypes"), "Mode"=TelemetryUpdateModes."=" ("TelemetryUpdateModes"), "Field"=TelemetryFields."InclinometerErrorCode", "Data"=InclinometerErrorCodes."SensorReportsIllegalFunction" ("InclinometerErrorCodes")) -> (w496:T10)
        n197 = xnode ("FIFO Method Node")("Element"=w496, "Timeout"=0) -> ()  [unwired: 1 in, 2 out]
        n198 = Bundle By Name(cluster=w504, "InclinometerState"=InclinometerStates."WaitForTrigger") -> (w505:T1)
      }
      frame "SensorReportsIllegalDataAddress" {
        n199 = call "GetTelemetryUpdateDataConstant.vi"() -> ("TelemetryUpdateData"=w511:T10)  [unwired: 11 in]
        n200 = Bundle By Name(cluster=w511, "DataType"=TelemetryDataTypes."U8" ("TelemetryDataTypes"), "Mode"=TelemetryUpdateModes."=" ("TelemetryUpdateModes"), "Field"=TelemetryFields."InclinometerErrorCode", "Data"=InclinometerErrorCodes."SensorReportsIllegalDataAddress" ("InclinometerErrorCodes")) -> (w506:T10)
        n201 = xnode ("FIFO Method Node")("Element"=w506, "Timeout"=0) -> ()  [unwired: 1 in, 2 out]
        n202 = Bundle By Name(cluster=w514, "InclinometerState"=InclinometerStates."WaitForTrigger") -> (w515:T1)
      }
    }
  }
  n203 = node-c288(w2) -> ()
